vi "Open acquisition file for write.vi"(7 "Number of acquisition files":i32, 8 "Existing directory to over-write":path, 9 "Use new?":bool, 10 "New directory to create":path) -> (0 "OK?":bool, 3 "Sequence files handle":T1)   [LabVIEW 2016]
uses:
  Sequence files handle.ctt
  GLIMPSE Globals.vi
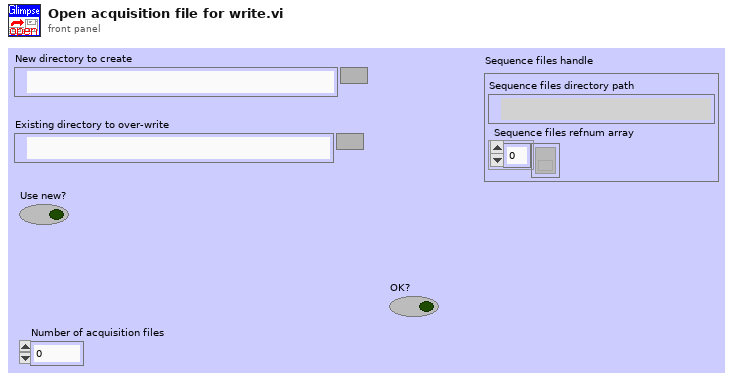
[diagram p1: front panel]
types:
  T1 = typedef "Sequence files handle.ctt" = cluster{"Sequence files directory path":path, "Sequence files refnum array":refnum<file>[]}
  T2 = enum16{"open", "replace", "create", "open or create", "replace or create", "replace or create with confirmation"}
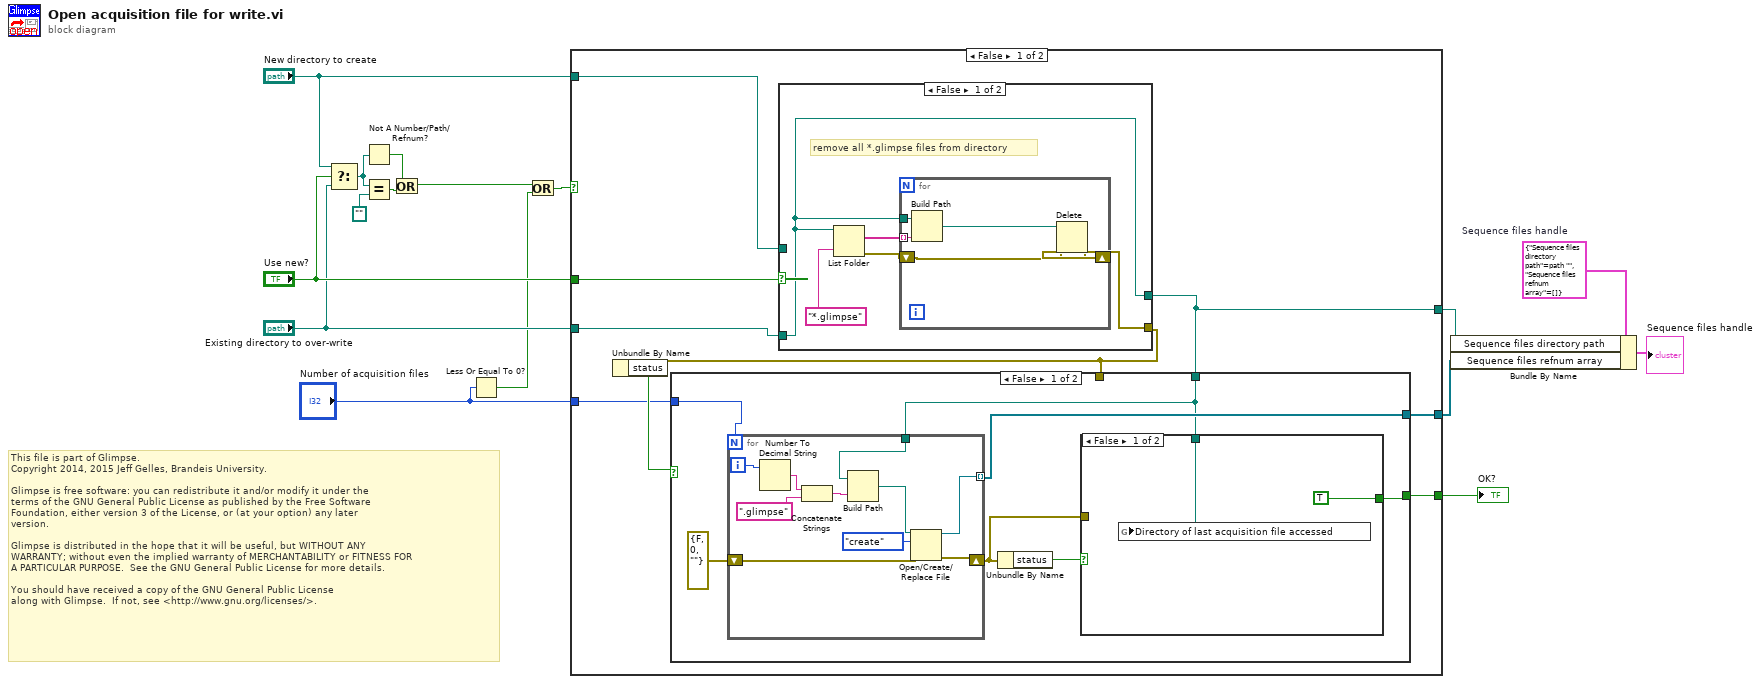
[diagram p0: block diagram]
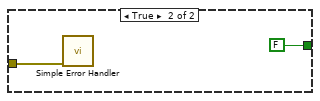
[diagram p2: hidden frame]
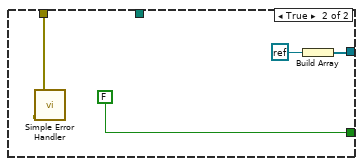
[diagram p3: hidden frame]
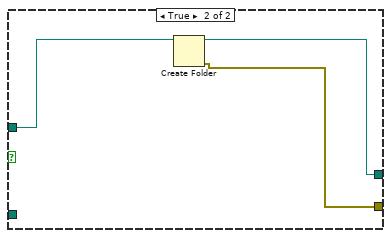
[diagram p4: hidden frame]
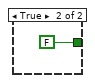
[diagram p5: hidden frame]
diagram:
  w1 = T1 {"Sequence files directory path"=path "", "Sequence files refnum array"=[]}  # Sequence files handle
  # "This file is part of Glimpse. \nCopyright 2014, 2015 Jeff Gelles, Brandeis University.    \n\nGlimpse is free software: you can redistribute it and/or modify it under the \nterms of the GNU General Public License as published by the Free Software \nFoundation, either version 3 of the License, or (at your option) any later \nversion.\n\nGlimpse is distributed in the hope that it will be useful, but WITHOUT ANY \nWARRANTY; without even the implied warranty of MERCHANTABILITY or FITNESS FOR \nA PARTICULAR PURPOSE.  See the GNU General Public License for more details.\n\nYou should have received a copy of the GNU General Public License\nalong with Glimpse.  If not, see <http://www.gnu.org/licenses/>."
  n1 = Select(t="New directory to create", s="Use new?", f="Existing directory to over-write") -> (s? t:f=w10:path)
  n2 = Not A Number/Path/Refnum?(number/path/refnum=w10) -> (NaN/Path/Refnum?=w9:bool)
  n3 = Equal?(x=w10, y=path "") -> (x = y?=w11:bool)
  n4 = Or(x=w9, y=w11) -> (x .or. y?=w8:bool)
  n5 = Less Or Equal To 0?(x="Number of acquisition files") -> (x <= 0?=w5:bool)
  n6 = Or(x=w8, y=w5) -> (x .or. y?=w7:bool)
  n7 = case shown="False" w7 {
    tunnel: [w23 FALSE] -> w16
    tunnel: [w22 _] -> w4
    tunnel: "Use new?" -> [w21 _]
    tunnel: "New directory to create" -> [w20 _]
    tunnel: "Existing directory to over-write" -> [w19 _]
    tunnel: "Number of acquisition files" -> [w18 _]
    tunnel: [w17 _] -> w3
    frame False {
      n8 = case shown="False" w21 {
        tunnel: [w51 w63] -> w17
        tunnel: [w52 w61] -> w25
        tunnel: w20 -> [_ w62]
        tunnel: w19 -> [w51 _]
        frame False {
          # "remove all *.glimpse files from directory"
          n9 = List Folder(path=w51, pattern="*.glimpse" ("name or relative path")) -> (filenames=w53:string[], error out=w54:errorcluster)  [unwired: 1 in, 3 out]
          n10 = for {
            shift-right: [w59] -> w52
            shift-left: w54 -> [w60]
            tunnel: w53 -> [w57] mode=indexing
            tunnel: w51 -> [w56]
            n11 = Build Path(base path=w56, name or relative path=w57) -> (appended path=w58:path)
            n12 = Delete(path (use dialog)=w58, error in=w60) -> (error out=w59:errorcluster)  [unwired: 5 out]
          }
        }
        frame True {
          n13 = Create Folder(path (use dialog)=w62) -> (created path=w63:path, error out=w61:errorcluster)  [unwired: 1 in, 2 out]
        }
      }
      n14 = Unbundle By Name(w25) -> ("status"=w24:bool)
      n15 = case shown="False" w24 {
        tunnel: w25 -> [_ w50]
        tunnel: w17 -> [w28 _]
        tunnel: [w31 FALSE] -> w23
        tunnel: [w29 w47] -> w22
        tunnel: w18 -> [w27 _]
        frame False {
          n16 = for {
            N: w27 -> [_]
            shift-right: [w38] -> w30
            shift-left: errorcluster {"status"=FALSE, "code"=0, "source"=""} ("error out") -> [w43]
            tunnel: w28 -> [w41]
            tunnel: [w39] -> w29 mode=indexing
            i -> [w46]
            n17 = Number To Decimal String(number=w46) -> (decimal integer string=w45:string)  [unwired: 1 out]
            n18 = Concatenate Strings(w45, ".glimpse" ("string")) -> (w42:string)
            n19 = Build Path(base path=w41, name or relative path=w42) -> (appended path=w40:path)
            n20 = Open/Create/Replace File(file path (use dialog)=w40, error in=w43, operation (0:open)=T2."create") -> (refnum out=w39:refnum<file>, error out=w38:errorcluster)  [unwired: 4 out]
          }
          n21 = Unbundle By Name(w30) -> ("status"=w32:bool)
          n22 = case shown="False" w32 {
            tunnel: [TRUE FALSE] -> w31
            tunnel: w30 -> [_ w35]
            tunnel: w28 -> [w33 _]
            frame False {
              n23 = global write "GLIMPSE Globals.vi" "Directory of last acquisition file accessed"(w33) -> ()
            }
            frame True {
              n24 = call <vilib>:"Simple Error Handler.vi"("error in (no error)"=w35) -> ()  [unwired: 1 in, 8 out]
            }
          }
        }
        frame True {
          n25 = call <vilib>:"Simple Error Handler.vi"("error in (no error)"=w50) -> ()  [unwired: 1 in, 8 out]
          n26 = Build Array(refnum<k0> refnum) -> (w47:refnum<k0>[])
        }
      }
    }
    frame True {
    }
  }
  "OK?" <- w16
  n27 = Bundle By Name(cluster=w1, "Sequence files directory path"=w3, "Sequence files refnum array"=w4) -> (→"Sequence files handle":T1)
